vi "Set Ramping Mode.vi"(2 "error in":T1, 3 "Ramping Mode":u16(ring) items=["RAMP", "PAUSE", "MANUAL UP", "MANUAL DOWN", "ZERO"], 4 "VISA resource name":refnum<visa-resource-name>) -> (0 "error out":T1, 1 "VISA resource name out":refnum<visa-resource-name>)   [LabVIEW 2019]
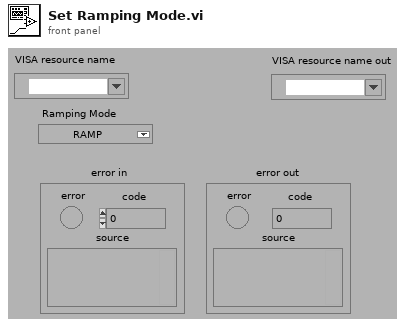
[diagram p1: front panel]
types:
  T1 = cluster{"error":bool, "code":i32, "source":string}
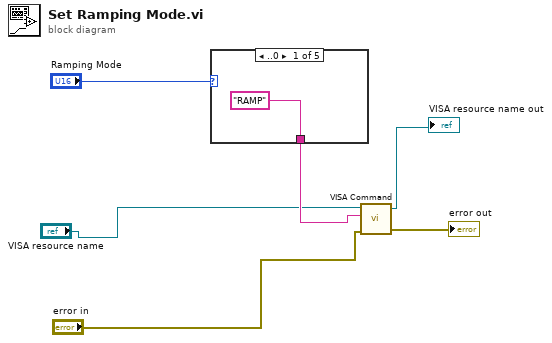
[diagram p0: block diagram]
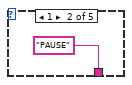
[diagram p2: hidden frame]
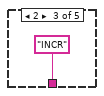
[diagram p3: hidden frame]
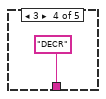
[diagram p4: hidden frame]
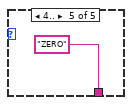
[diagram p5: hidden frame]
diagram:
  n1 = case shown="..0" "Ramping Mode" {
    tunnel: ["RAMP" "PAUSE" "INCR" "DECR" "ZERO"] -> w5
    frame ..0 {
    }
    frame 1 {
    }
    frame 2 {
    }
    frame 3 {
    }
    frame 4.. {
    }
  }
  n2 = call "VISA Command.vi"("error in (no error)"="error in", "Command"=w5, "VISA resource name"="VISA resource name") -> ("error out"=→"error out":errorcluster, "VISA resource name out"=→"VISA resource name out":refnum<visa-resource-name>)  [unwired: 1 in, 1 out]
